vi "NI VeriStand - Load Runtime Configuration File.vi"(8 "Error in":errorcluster, 11 "Runtime Configuration File":string) -> (0 "Error out":errorcluster, 3 "Runtime Configuration Ref":refnum<k24>)   [LabVIEW 2025, in "NI_VS RuntimeConfigurationFile ScriptingAPI.lvlib"]
uses:
  NI_VS RuntimeConfigurationFile ScriptingAPI.lvlib
  NationalInstruments.VeriStand.SystemDefinitionAPI
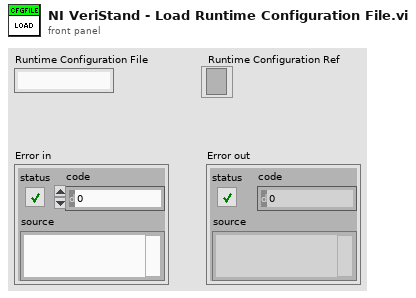
[diagram p1: front panel]
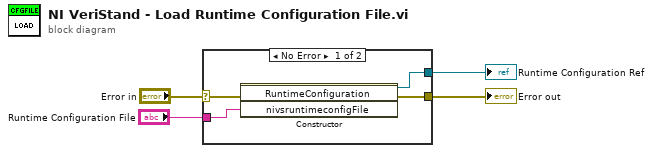
[diagram p0: block diagram]
diagram:
  n1 = case shown="No Error" "Error in" {
    selector: "Error in" -> [w8 w9]
    tunnel: [w6 _] -> w2
    tunnel: [w7 w9] -> w3
    tunnel: "Runtime Configuration File" -> [w5 _]
    frame No Error {
      n2 = constructor class="RuntimeConfiguration"(error in=w8, "nivsruntimeconfigFile"=w5) -> (reference out=w6:refnum<k24>, error out=w7:errorcluster)  [unwired: 2 in, 2 out]
    }
    frame Error {
    }
  }
  "Error out" <- w3
  "Runtime Configuration Ref" <- w2
